vi "CheckFileName.vi"(8 "Error In":errorcluster, 11 "File Name in":string) -> (0 "Error Out":errorcluster, 3 "File Name out":string)   [LabVIEW 2018, in "AcPwrPlugins.lvlib" / "AcPwrBase.lvclass"]
doc: "Checks the file name for a .ini file extension and adds one if not present. If a different file extension is present this VI will strip it and add a .ini file extension."
uses:
  AcPwrBase.lvclass
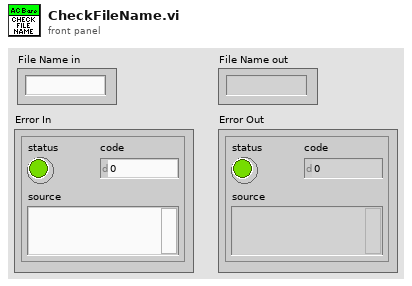
[diagram p1: front panel]
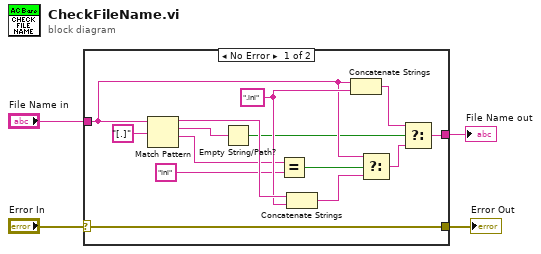
[diagram p0: block diagram]
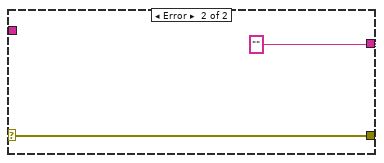
[diagram p2: hidden frame]
diagram:
  n1 = case shown="No Error" "Error In" {
    selector: "Error In" -> [w5 w19]
    tunnel: "File Name in" -> [w10 _]
    tunnel: [w8 "" ("File Name in")] -> w3
    tunnel: [w5 w19] -> w1
    frame No Error {
      w16 = ".ini" ("string")
      n2 = Match Pattern(string=w10, regular expression="[.]" ("string")) -> (before substring=w17:string, match substring=w13:string, after substring=w14:string)  [unwired: 1 in, 1 out]
      n3 = Empty String/Path?(string/path=w13) -> (empty?=w6:bool)
      n4 = Equal?(x=w14, y="ini" ("string")) -> (x = y?=w9:bool)
      n5 = Concatenate Strings(w17, w16) -> (w18:string)
      n6 = Concatenate Strings(w10, w16) -> (w7:string)
      n7 = Select(t=w10, s=w9, f=w18) -> (s? t:f=w11:string)
      n8 = Select(t=w7, s=w6, f=w11) -> (s? t:f=w8:string)
    }
    frame Error {
    }
  }
  "File Name out" <- w3
  "Error Out" <- w1
